vi "IsMotorPosWithinRange.vi"(8 "Which axis?":T1, 9 "Allowed difference":T2, 10 "Wanted Position":T2, 11 "Current Position":T2) -> (3 "In range?":bool)   [LabVIEW 2011]
uses:
  MotorPosType.ctl
  Typedefs/XYf.ctl
  MotorPosFlagsType.ctl
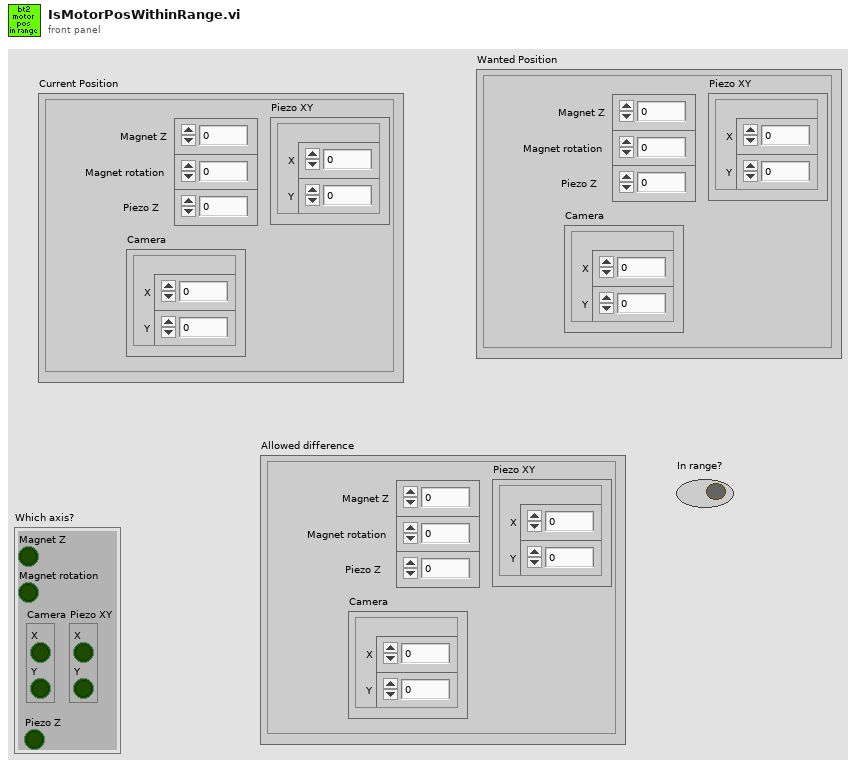
[diagram p1: front panel]
types:
  T1 = typedef "MotorPosFlagsType.ctl" = cluster{"Magnet Z":bool, "Magnet rotation":bool, "Camera":cluster{"X":bool, "Y":bool}, "Piezo XY":cluster{"X":bool, "Y":bool}, "Piezo Z":bool}
  T2 = typedef "MotorPosType.ctl" = cluster{"Magnet Z":dbl, "Magnet rotation":dbl, "Camera":T3, "Piezo XY":T3, "Piezo Z":dbl}
  T3 = typedef "XYf.ctl" = cluster{"X":sgl, "Y":sgl}
  T4 = cluster{"Magnet Z":bool, "Magnet rotation":bool, "Camera":cluster{"X":bool, "Y":bool}, "Piezo XY":cluster{"X":bool, "Y":bool}, "Piezo Z":bool}
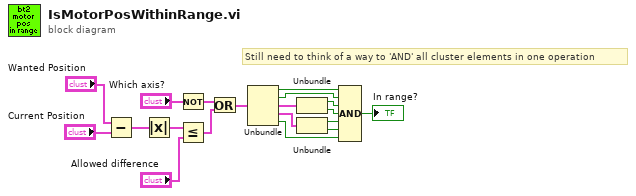
[diagram p0: block diagram]
diagram:
  # "Still need to think of a way to 'AND' all cluster elements in one operation"
  n1 = Subtract(x="Wanted Position", y="Current Position") -> (x-y=w17:T2)
  n2 = Absolute Value(x=w17) -> (abs(x)=w16:T2)
  n3 = Not(x="Which axis?") -> (.not. x?=w13:T1)
  n4 = Less Or Equal?(x=w16, y="Allowed difference") -> (x <= y?=w12:T4)
  n5 = Or(x=w13, y=w12) -> (x .or. y?=w11:T1)
  n6 = Unbundle(w11) -> ("Magnet Z"=w8:bool, "Magnet rotation"=w7:bool, "Camera"=w10:cluster{"X":bool, "Y":bool}, "Piezo XY"=w9:cluster{"X":bool, "Y":bool}, "Piezo Z"=w2:bool)
  n7 = Unbundle(w10) -> ("X"=w6:bool, "Y"=w5:bool)
  n8 = Unbundle(w9) -> ("X"=w4:bool, "Y"=w3:bool)
  n9 = Compound Arithmetic op=AND(w8, w7, w6, w5, w4, w3, w2) -> (→"In range?":bool)
